vi "test Create and Delete Container.vi"(8 "error in (no error)":errorcluster, 11 "TestCase in":refnum<class "Test_Blob.lvclass">) -> (0 "error out":errorcluster, 3 "TestCase out":refnum<class "Test_Blob.lvclass">)   [LabVIEW 2015, in "Test_Blob.lvclass"]
uses:
  Test_Blob.lvclass
  Global Parameters.vi
  Core/Session/Session.lvclass
  Blob Storage/NI_Azure_Blob.lvlib
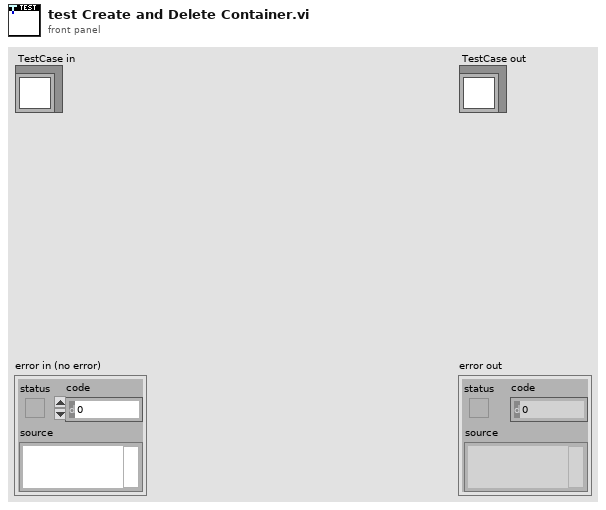
[diagram p1: front panel]
types:
  T1 = typedef "NI_Azure_Core.lvlib/Session.lvclass/Azure Credentials.ctl" = cluster{"Storage Account Name":string, "Access Key":string}
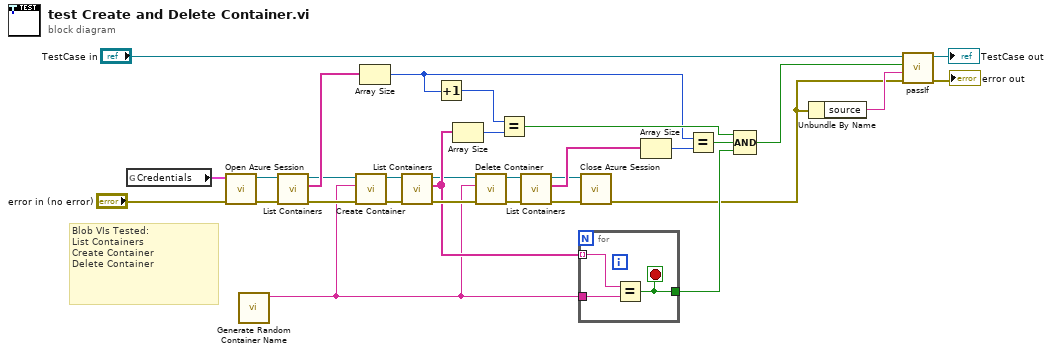
[diagram p0: block diagram]
diagram:
  # "Blob VIs Tested:\nList Containers\nCreate Container\nDelete Container"
  n1 = global read "Global Parameters.vi" "Credentials"() -> (w12:T1)
  n2 = call "Open Azure Session.vi"("error in (no error)"="error in (no error)", "Credentials"=w12) -> ("error out"=w15:errorcluster, "Azure Session"=w11:refnum<class "Session.lvclass">)  [unwired: 8 in]
  n3 = call "Generate Random Container Name.vi"() -> ("Random Container Name"=w5:string)  [unwired: 11 in]
  n4 = call "List Containers.vi"("error in (no error)"=w15, "Azure Session in"=w11) -> ("error out"=w27:errorcluster, "Containers"=w10:string[], "Azure Session out"=w9:refnum<class "Session.lvclass">)  [unwired: 7 in]
  n5 = call "Create Container.vi"("error in (no error)"=w27, "Container"=w5, "Azure Session in"=w9) -> ("error out"=w26:errorcluster, "Azure Session out"=w8:refnum<class "Session.lvclass">)  [unwired: 7 in]
  n6 = Array Size(array=w10) -> (size(s)=w19:i32)
  n7 = call "List Containers.vi"("error in (no error)"=w26, "Azure Session in"=w8) -> ("error out"=w25:errorcluster, "Containers"=w7:string[], "Azure Session out"=w6:refnum<class "Session.lvclass">)  [unwired: 7 in]
  n8 = Increment(x=w19) -> (x+1=w22:i32)
  n9 = Array Size(array=w7) -> (size(s)=w23:i32)
  n10 = call "Delete Container.vi"("error in (no error)"=w25, "Container"=w5, "Azure Session in"=w6) -> ("error out"=w24:errorcluster, "Azure Session out"=w4:refnum<class "Session.lvclass">)  [unwired: 7 in]
  n11 = Equal?(x=w22, y=w23) -> (x = y?=w21:bool)
  n12 = call "List Containers.vi"("error in (no error)"=w24, "Azure Session in"=w4) -> ("error out"=w13:errorcluster, "Containers"=w3:string[], "Azure Session out"=w1:refnum<class "Session.lvclass">)  [unwired: 7 in]
  n13 = for {
    tunnel: w7 -> [w34] mode=indexing
    tunnel: w5 -> [w33]
    tunnel: [w32] -> w17
    stop <- w32 stop-if-true
    n14 = Equal?(x=w34, y=w33) -> (x = y?=w32:bool)
  }
  n15 = call "Close Azure Session.vi"("error in (no error)"=w13, "Azure Session"=w1) -> ("error out"=w2:errorcluster)  [unwired: 9 in]
  n16 = Array Size(array=w3) -> (size(s)=w20:i32)
  n17 = Equal?(x=w19, y=w20) -> (x = y?=w18:bool)
  n18 = Compound Arithmetic op=AND(w21, w18, w17) -> (w16:bool)
  n19 = Unbundle By Name(w2) -> ("source"=w28:string)
  n20 = call-dynamic "passIf.vi"("error in (no error)"=w2, "message (\"\")"=w28, "pass"=w16, "TestCase in"="TestCase in") -> ("error out"=→"error out":errorcluster, "TestCase out"=→"TestCase out":refnum<class "Test_Blob.lvclass">)  [unwired: 6 in]
